vi "Close Interlocks.vi"(8 "error in (no error)":errorcluster, 9 "Interlock? (F)":bool, 11 "Interlocks in":refnum<class "Interlock.lvclass">[](array[class])) -> (0 "error out":errorcluster, 3 "Interlocks out":refnum<class "Interlock.lvclass">[](array[class]))   [LabVIEW 2015, in "Interlocks.lvlib" / "Interlock.lvclass"]
uses:
  Interlock.lvclass
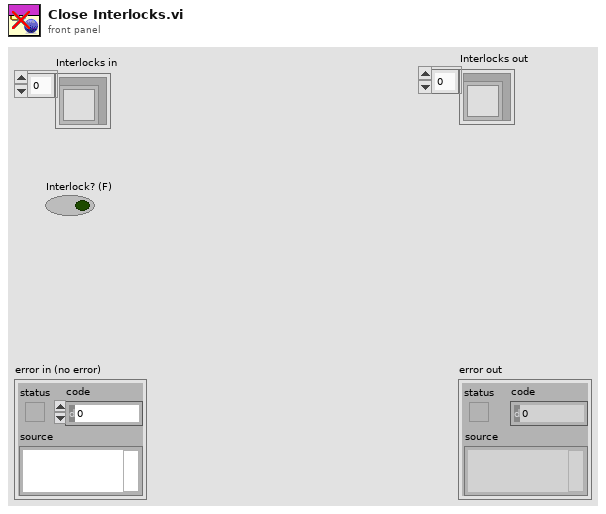
[diagram p1: front panel]
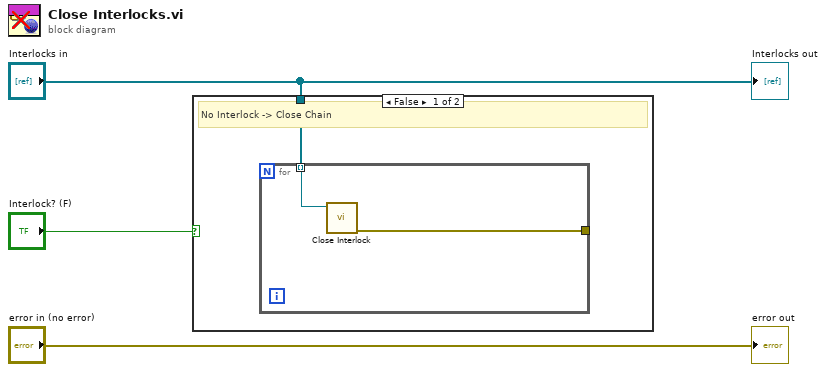
[diagram p0: block diagram]
diagram:
  n1 = case shown="False" "Interlock? (F)" {
    tunnel: "Interlocks in" -> [w4 _]
    frame False {
      # "No Interlock -> Close Chain"
      n2 = for {
        tunnel: w4 -> [w6] mode=indexing
        tunnel: [w5] -> _
        n3 = call-dynamic "Close Interlock.vi"("Interlock in"=w6) -> ("error out"=w5:errorcluster)  [unwired: 9 in, 1 out]
      }
    }
    frame True {
      # "Interlock -> Keep connections open"
    }
  }
  "error out" <- "error in (no error)"
  "Interlocks out" <- "Interlocks in"
